vi "merFISH_move_to_XY_position.vi"(5 "ROI #":i32, 6 "Global parameters":T1 {"# repetitions" min=0; "Dt (s)" min=0 step=1; "Filter list" items=["ET665lp", "zet405/488/561/640m", "None", "None", "None", "None"]}, 8 "queue ASI stage":refnum<queue>, 10 "error in":errorcluster, 11 "XY positions":dbl[][](array[numeric])) -> (0 "Global parameters out":T1 {"# repetitions" min=0; "Dt (s)" min=0 step=1; "Filter list" items=["ET665lp", "zet405/488/561/640m", "None", "None", "None", "None"]}, 1 "error out":errorcluster, 3 "XY positions":dbl[][](array[numeric]))   [LabVIEW 2015]
uses:
  CONTROLS/Global parameters.ctl
  CONTROLS/Q_ASI_stage_element.ctl
  GLOBAL/Global_ASI_stage.vi
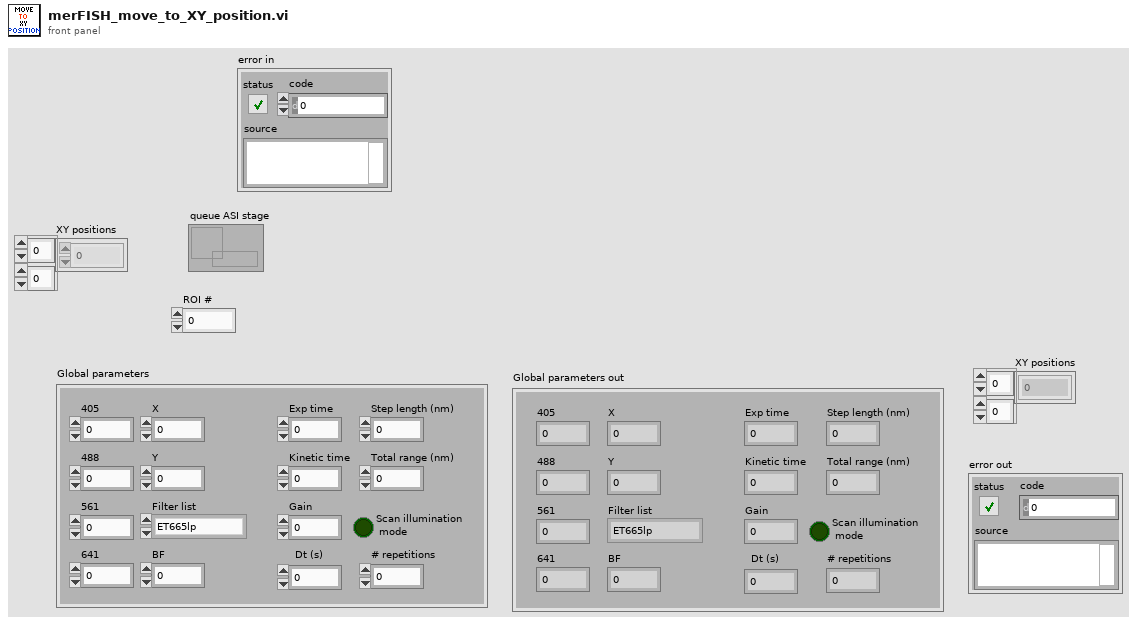
[diagram p1: front panel]
types:
  T1 = typedef "Global parameters.ctl" = cluster{"405":dbl, "488":dbl, "561":dbl, "641":dbl, "BF":dbl, "X":dbl, "Y":dbl, "Filter list":u16, "Exp time":sgl, "Kinetic time":sgl, "Gain":i32, "Step length (nm)":u32, "Total range (nm)":u32, "Scan illumination\n mode":bool, "Dt (s)":i32, "# repetitions":i32}
  T2 = typedef "Q_ASI_stage_element.ctl" = cluster{"variant":variant, "Instruction":enum16{"ASI_idle", "ASI_initialize", "ASI_error", "ASI_security_stop", "ASI_read_XYZ", "ASI_up", "ASI_down", "ASI_left", "ASI_right", "ASI_save_XY", "ASI_move_to_XY", "ASI_brightfield", "ASI_init_scan", "ASI_init_merFISH", "ASI_move_to_XY_merFISH", "ASI_move_to_Z_merFISH", "ASI_init_autofocus_search_merFISH", "ASI_close_autofocus_search_merFISH", "ASI_adjust_piezo_autofocus_merFISH", "ASI_set_piezo_autofocus_to_reference_position_merFISH_TL", "ASI_close_merFISH", "ASI_stop"}}
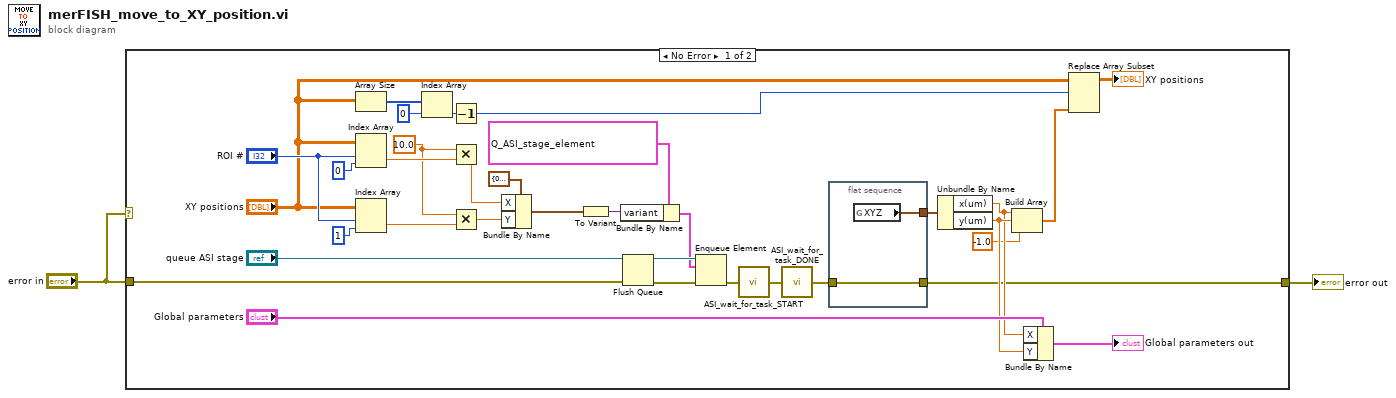
[diagram p0: block diagram]
diagram:
  n1 = case shown="No Error" "error in" {
    tunnel: "error in" -> [w25 w39]
    tunnel: [w6 w39] -> w2
    frame No Error {
      w27 = 10.0
      n2 = Array Size(array="XY positions") -> (size(s)=w35:i32[])
      n3 = Index Array(array="XY positions", index (row)="ROI #", index (col)=0 ("disabled index (col)")) -> (element=w28:dbl)
      n4 = Index Array(array="XY positions", index (row)="ROI #", index (col)=1 ("disabled index (col)")) -> (element=w29:dbl)
      n5 = Index Array(array=w35, index=0) -> (element=w33:i32)
      n6 = Decrement(x=w33) -> (x-1=w32:i32)
      n7 = Multiply(x=w27, y=w28) -> (x*y=w17:dbl)
      n8 = Multiply(x=w27, y=w29) -> (x*y=w16:dbl)
      n9 = Bundle By Name(cluster=cluster{"X":dbl, "Y":dbl} {"X"=0.0, "Y"=0.0} ("output cluster"), "X"=w17, "Y"=w16) -> (w4:cluster{"X":dbl, "Y":dbl})
      n10 = To Variant(anything=w4) -> (Variant=w21:variant)
      n11 = Bundle By Name(cluster=T2 {"variant"=variant, "Instruction"=enum."ASI_move_to_XY_merFISH"} ("Q_ASI_stage"), "variant"=w21) -> (w20:T2)
      n12 = Flush Queue(queue="queue ASI stage", error in (no error)=w25) -> (queue out=w23:refnum<queue>, error out=w24:errorcluster)  [unwired: 1 out]
      n13 = Enqueue Element(queue=w23, element=w20, error in (no error)=w24) -> (error out=w19:errorcluster)  [unwired: 1 in, 2 out]
      n14 = call "ASI_wait_for_task_START.vi"("error in"=w19) -> ("error out"=w18:errorcluster)
      n15 = call "ASI_wait_for_task_DONE.vi"("error in"=w18) -> ("error out"=w15:errorcluster)
      n16 = flat-sequence {
        tunnel: w15 -> [w38]
        tunnel: [w38] -> w6
        tunnel: [w37] -> w14
        frame #0 {
          n17 = global read "Global_ASI_stage.vi" "XYZ"() -> (w37:cluster{"x(um)":dbl, "y(um)":dbl, "z(um)":dbl})
        }
      }
      n18 = Unbundle By Name(w14) -> ("x(um)"=w11:dbl, "y(um)"=w12:dbl)
      n19 = Build Array(w11, w12, -1.0 ("element")) -> (w36:dbl[])
      n20 = Bundle By Name(cluster="Global parameters", "X"=w11, "Y"=w12) -> (→"Global parameters out":T1)
      n21 = Replace Array Subset(array="XY positions", new element=w36, index (row)=w32) -> (→"XY positions":dbl[][])  [unwired: 1 in]
    }
    frame Error {
    }
  }
  "error out" <- w2
